vi "Test-Host-Step-3.vi"() -> ()   [LabVIEW 2017]
panel:
  out "size(hp_state-u64)":i32
  out "size(hp_state)":i32
  out "hp_state_out (u64)":u64[](array[numeric]) format="%.0x"
  out "exp_hp_state_out (u64)":u64[](array[numeric]) format="%.0x"
  out "Values Match?":bool
  out "exp_hp_state_out":u8[](array[numeric]) format="%.0x"
  out "Runtime (minutes)":dbl
  in  "Override Iterations":bool
  out "Runtime (s)":dbl
  out "Runtime (ms)":u32
  in  "# of Iterations":i32=1
  out "b_out":u64[](array[numeric]) format="%.0x"
  out "a_out":u64[](array[numeric]) format="%.0x"
  in  "FileName":string="log_file.8.bin"
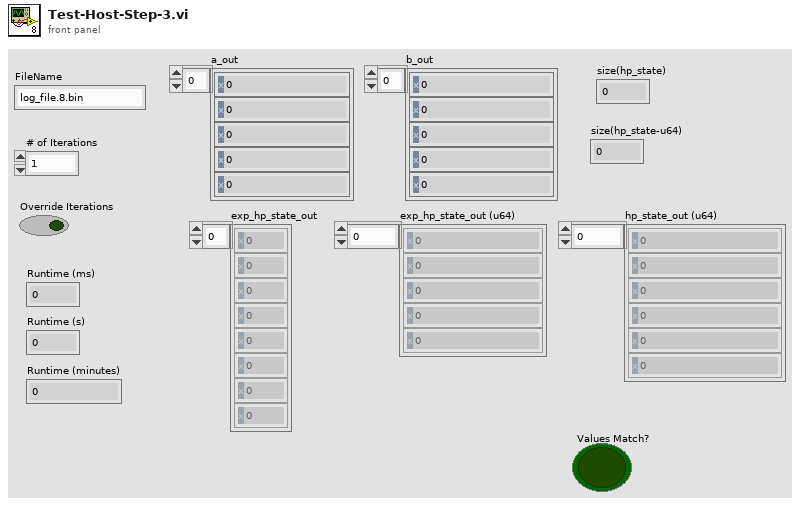
[diagram p1: front panel]
types:
  T1 = typedef "Step-3-Data-Type.ctl" = cluster{"a":u64[], "b":u64[], "hp_state_in":u8[], "hp_state_out":u8[], "hp_state_in (u64)":u64[], "hp_state_out (u64)":u64[]}
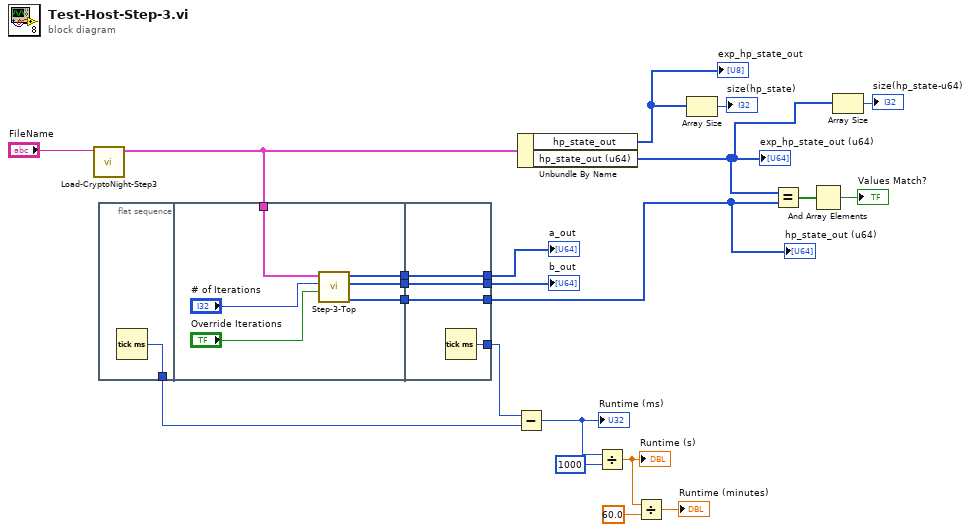
[diagram p0: block diagram]
diagram:
  n1 = call "Load-CryptoNight-Step3.vi"("FileName"="FileName") -> ("output cluster"=w10:T1)  [unwired: 9 in, 1 out]
  n2 = flat-sequence {
    tunnel: [w22] -> w16
    tunnel: [w28] -> w19
    tunnel: [w27] -> w18
    tunnel: w10 -> [w24]
    tunnel: [w23] -> w8
    tunnel: [w31] -> w20
    tunnel: [w32] -> w21
    tunnel: w19 -> [w32]
    tunnel: w18 -> [w31]
    tunnel: [w30] -> w17
    tunnel: [w29] -> w5
    tunnel: w8 -> [w29]
    frame #0 {
      n3 = Tick Count (ms)() -> (millisecond timer value=w22:u32)
    }
    frame #1 {
      n4 = call "Step-3-Top.vi"("Override Iterations"="Override Iterations", "# of Iterations"="# of Iterations", "input"=w24) -> ("hp_state out (u64)"=w23:u64[], "b_out"=w27:u64[], "a_out"=w28:u64[])  [unwired: 6 in]
    }
    frame #2 {
      n5 = Tick Count (ms)() -> (millisecond timer value=w30:u32)
    }
  }
  n6 = Subtract(x=w17, y=w16) -> (x-y=w15:u32)
  "Runtime (ms)" <- w15
  n7 = Unbundle By Name(w10) -> ("hp_state_out"=w4:u8[], "hp_state_out (u64)"=w1:u64[])
  "exp_hp_state_out" <- w4
  "exp_hp_state_out (u64)" <- w1
  n8 = Divide(x=w15, y=u32 1000) -> (x/y=w13:dbl)
  "Runtime (s)" <- w13
  n9 = Divide(x=w13, y=60.0) -> (x/y=→"Runtime (minutes)":dbl)
  n10 = Array Size(array=w4) -> (size(s)=→"size(hp_state)":i32)
  n11 = Equal?(x=w1, y=w5) -> (x = y?=w7:bool[])
  n12 = And Array Elements(Boolean array=w7) -> (logical AND=→"Values Match?":bool)
  n13 = Array Size(array=w1) -> (size(s)=→"size(hp_state-u64)":i32)
  "a_out" <- w21
  "b_out" <- w20
  "hp_state_out (u64)" <- w5
